vi "Check Mainframe.vi"(8 "error in":errorcluster, 10 "Mainframe":i32=1, 11 "VISA resource name":refnum<visa-resource-name>) -> (0 "error out":errorcluster, 2 "Version Output":string, 3 "VISA resource name out":refnum<visa-resource-name>)   [LabVIEW 2018]
panel:
  out "Mainframe Output":string
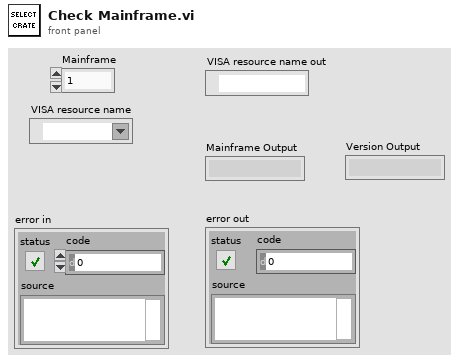
[diagram p1: front panel]
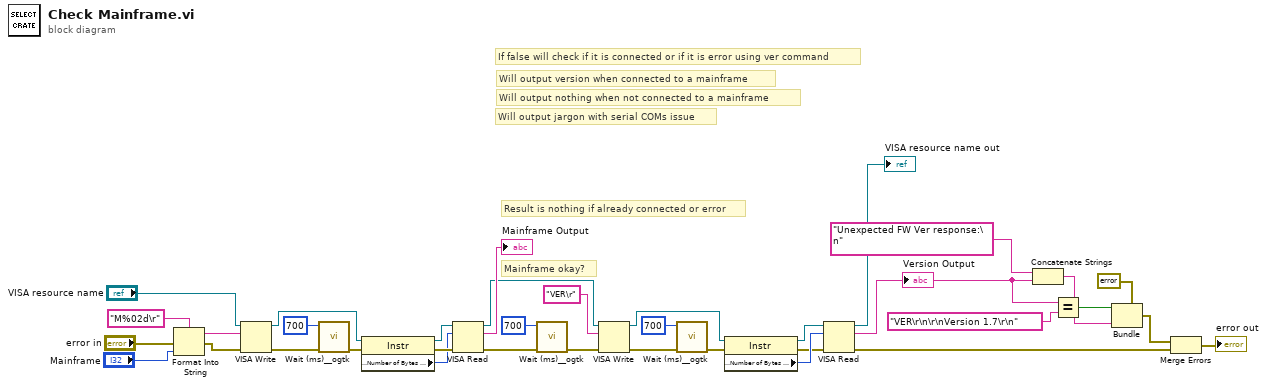
[diagram p0: block diagram]
diagram:
  # "Will output jargon with serial COMs issue"
  # "Will output nothing when not connected to a mainframe"
  # "Will output version when connected to a mainframe"
  # "If false will check if it is connected or if it is error using ver command"
  # "Mainframe okay?"
  # "Result is nothing if already connected or error"
  n1 = Format Into String(format string="M%02d\r", error in="error in", "Mainframe") -> (resulting string=w2:string, error out=w1:errorcluster)  [unwired: 1 in]
  n2 = VISA Write(VISA resource name="VISA resource name", write buffer=w2, error in (no error)=w1) -> (VISA resource name out=w30:refnum<visa-resource-name>, error out=w35:errorcluster)  [unwired: 1 out]
  n3 = call <userlib>:"Wait (ms)__ogtk.vi"("error in (no error)"=w35, "milliseconds to wait"=u32 700) -> ("error out"=w29:errorcluster)  [unwired: 8 in, 1 out]
  n4 = property class="Instr"(reference=w30, error in=w29) -> (reference out=w32:refnum<visa-resource-name>, error out=w33:errorcluster, "Serial Settings:Number of Bytes at Serial Port"=w31:u32)
  n5 = VISA Read(VISA resource name=w32, byte count=w31, error in (no error)=w33) -> (VISA resource name out=w27:refnum<visa-resource-name>, read buffer=→"Mainframe Output":string, error out=w25:errorcluster)  [unwired: 1 out]
  n6 = call <userlib>:"Wait (ms)__ogtk.vi"("error in (no error)"=w25, "milliseconds to wait"=u32 700) -> ("error out"=w24:errorcluster)  [unwired: 8 in, 1 out]
  n7 = VISA Write(VISA resource name=w27, write buffer="VER\r", error in (no error)=w24) -> (VISA resource name out=w21:refnum<visa-resource-name>, error out=w17:errorcluster)  [unwired: 1 out]
  n8 = call <userlib>:"Wait (ms)__ogtk.vi"("error in (no error)"=w17, "milliseconds to wait"=u32 700) -> ("error out"=w22:errorcluster)  [unwired: 8 in, 1 out]
  n9 = property class="Instr"(reference=w21, error in=w22) -> (reference out=w19:refnum<visa-resource-name>, error out=w18:errorcluster, "Serial Settings:Number of Bytes at Serial Port"=w20:u32)
  n10 = VISA Read(VISA resource name=w19, byte count=w20, error in (no error)=w18) -> (VISA resource name out=→"VISA resource name out":refnum<visa-resource-name>, read buffer=w6:string, error out=w11:errorcluster)  [unwired: 1 out]
  "Version Output" <- w6
  n11 = Concatenate Strings("Unexpected FW Ver response:\n", w6) -> (w7:string)
  n12 = Equal?(x=w6, y="VER\r\n\r\nVersion 1.7\r\n") -> (x = y?=w12:bool)
  n13 = Bundle(cluster=errorcluster {"status"=FALSE, "code"=0, "source"=""} ("error out"), "status"=w12, "source"=w7) -> (w10:errorcluster)  [unwired: 1 in]
  n14 = Merge Errors(w10, w11) -> (→"error out":errorcluster)
